vi "compare.compress.buffer.results.vi"(9 "buffer.length.out":u8, 10 "buffer.out":u64[](array[numeric])=[0, 0, 0, 0, 0, 0, 0, 0, 0] format="%.0x", 11 "Test Case":T1={"buffer"=[0, 0, 0, 0, 0, 0, 0, 0, 0], "buffer.length"=0, "start.idx"=0, "exp.buffer.length"=0, "exp.buffer"=[0, 0, 0, 0, 0, 0, 0, 0, 0]} {"exp.buffer" format="%.0x"; "buffer" format="%.0x"}) -> (1 "buffer elements":bool[](array[boolean]), 2 "length matches?":bool, 3 "Passed?":bool)   [LabVIEW 2020]
uses:
  compress.buffer.test.case.ctl
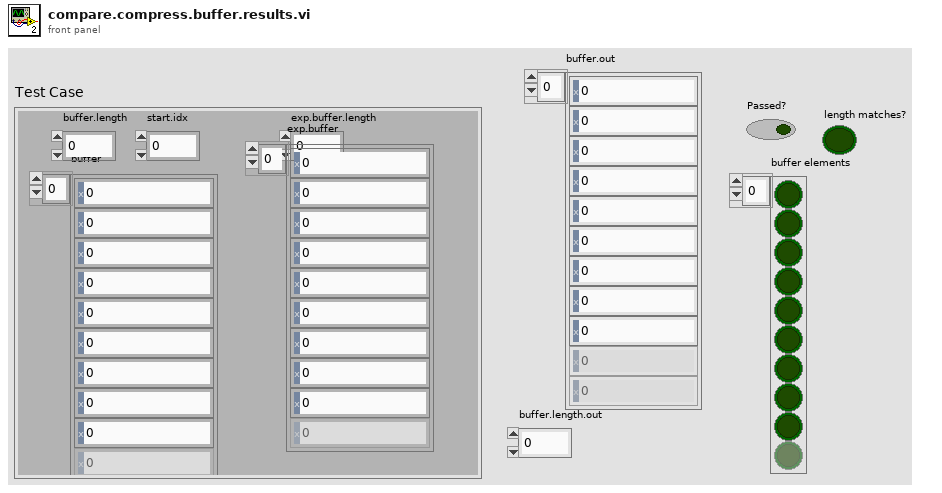
[diagram p1: front panel]
types:
  T1 = typedef "compress.buffer.test.case.ctl" = cluster{"buffer":u64[], "buffer.length":u8, "start.idx":u8, "exp.buffer.length":u8, "exp.buffer":u64[]}
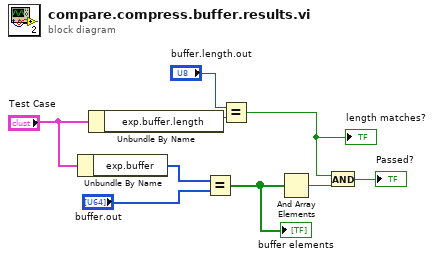
[diagram p0: block diagram]
diagram:
  n1 = Unbundle By Name("Test Case") -> ("exp.buffer"=w5:u64[])
  n2 = Unbundle By Name("Test Case") -> ("exp.buffer.length"=w8:u8)
  n3 = Equal?(x=w5, y="buffer.out") -> (x = y?=w3:bool[])
  "buffer elements" <- w3
  n4 = Equal?(x="buffer.length.out", y=w8) -> (x = y?=w7:bool)
  "length matches?" <- w7
  n5 = And Array Elements(Boolean array=w3) -> (logical AND=w2:bool)
  n6 = And(x=w7, y=w2) -> (x .and. y?=→"Passed?":bool)
